vi "flatten.vi"(8 "error in":errorcluster, 11 "test-group-legacy in":refnum<class " test-group-legacy.lvclass">) -> (0 "error out":errorcluster, 2 "flattened group":string, 3 "test-group-legacy out":refnum<class " test-group-legacy.lvclass">)   [LabVIEW 2020, in " test-group-legacy.lvclass"]
uses:
   test-group-legacy.lvclass
   test-group-legacy.lvclass/ test-group-legacy.ctl
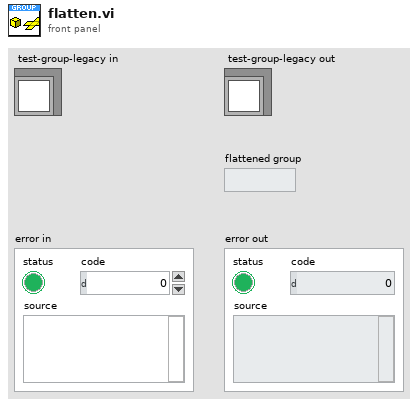
[diagram p1: front panel]
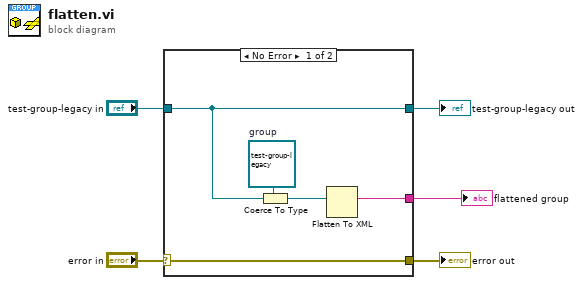
[diagram p0: block diagram]
diagram:
  n1 = case shown="No Error" "error in" {
    selector: "error in" -> [w10 w12]
    tunnel: [w10 w12] -> w4
    tunnel: [w8 w11] -> w2
    tunnel: "test-group-legacy in" -> [w8 w11]
    tunnel: [w9 _] -> w1
    frame No Error {
      w7 = refnum<class " test-group-legacy.lvclass"> refnum  # group
      n2 = Coerce To Type(0:w8, 1:w7) -> (2:w6:refnum<class " test-group-legacy.lvclass">)
      n3 = Flatten To XML(6:w6) -> (2:w9:string)
    }
    frame Error {
    }
  }
  "error out" <- w4
  "test-group-legacy out" <- w2
  "flattened group" <- w1
